vi "En Face Functional Global.vi"(8 "Error In":errorcluster, 10 "BScan Index":dbl, 11 "Input":sgl[][](graph)) -> (0 "Error Out":errorcluster)   [LabVIEW 2015]
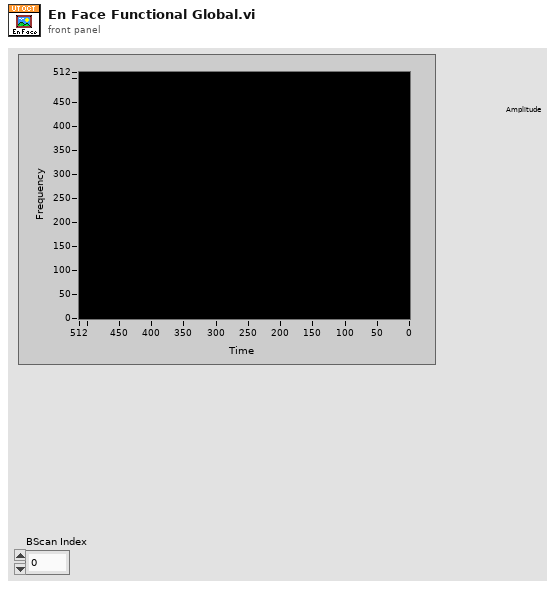
[diagram p1: front panel]
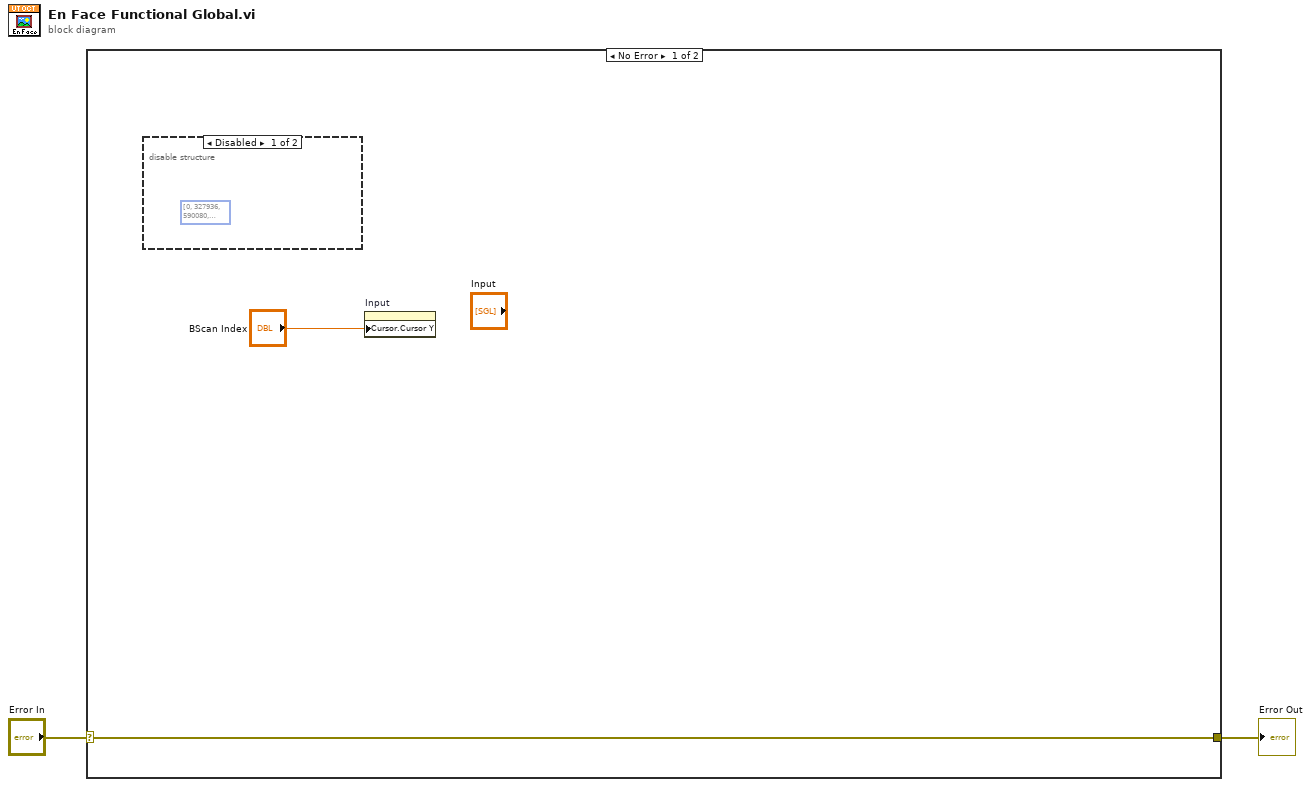
[diagram p0: block diagram]
diagram:
  n1 = case shown="No Error" "Error In" {
    selector: "Error In" -> [w4 w5]
    tunnel: [w4 w5] -> w1
    frame No Error {
      n2 = disable-structure shown="Disabled" {
        frame Disabled {
          (unwired) u32[] [0, 327936, 590080, 852224, 983296, 1114624, 1180160, 1311232, 1442304, 1573632, 1704704, 1770240, 1901312, 1966848, 2098176, 2163712, 2294784, 2491392, 2557184, 2688256, 2753792, 2884864, 2950656, 3081728, 3147264, 3344129, 3475457, 3540993, 3672321, 3738113, 3869185, 3934977, 4066305, 4197633, 4328961, 4394497, 4460289, 4591617, 4657409, 4788481, 4854273, 4985601, 5116929, 5248257, 5314049, 5379841, 5511169, 5576961, 5708033, 5773825, 5905153, 6036482, 6167810, 6233346, 6299138, 6430466, 6496258, 6562050, 6693634, 6759426, 6890754, 7022082, 7087874, 7153666, 7284994, 7350786, 7482114, 7547906, 7613698, 7745026, 7876354, 8007682, 8073474, 8139522, 8205314, 8336642, 8467970, 8533763, 8599555, 8665347, 8731139, 8862467, 8993795, 9059587, 9125380, 9191428, 9257220, 9388548, 9454340, 9520132, 9585924, 9717253, 9848837, 9914629, 9980165, 10045957, 10177541, 10243334, 10309126, 10375174, 10440966, 10572294, 10703623, 10769416, 10835208, 10901256, 10967049, 11033097, 11033609, 11099401, 11165450, 11231242, 11231754, 11297547, 11363339, 11429131, 11495180, 11495692, 11561740, 11693069, 11758861, 11759373, 11825165, 11891214, 11957006, 12022799, 12023311, 12089103, 12220944, 12286736, 12286736, 12352529, 12418577, 12484370, 12550162, 12615954, 12681747, 12747796, 12813588, 12813845, 12879894, 12945686, 13077015, 13142808, 13143064, 13208856, 13274905, 13340697, 13340953, 13472282, 13538075, 13604379, 13670172, 13735964, 13801757, 13867550, 13933343, 13999392, 13999648, 14065441, 14131234, 14197027, 14197541, 14263334, 14329383, 14395176, 14460969, 14592553, 14658346, 14724139, 14789932, 14790189, 14856238, 14922287, 14988080, 15053873, 15054130, 15119923, 15185972, 15251765, 15317559, 15383353, 15449146, 15449660, 15515454, 15515968, 15516226, 15582021, 15582278, 15582536, 15648587, 15648844, 15714639, 15714897, 15715155, 15780949, 15781463, 15847256, 15847770, 15848028, 15913823, 15914081, 15979875, 15980133, 15980391, 16046441, 16046444, 16046703, 16046705, 16112500, 16113015, 16113274, 16113277, 16179072, 16179330, 16179588, 16245384, 16245387, 16245389, 16245648, 16311443, 16376982, 16377241, 16377499, 16443294, 16443553, 16443555, 16443815, 16509866, 16510124, 16510127, 16575923, 16575924, 16576182, 16576441, 16576443, 16576702, 16576705, 16576963, 16577222, 16577224, 16577482, 16577485, 16577743, 16577745, 16578004, 16578262, 16578264, 16578523, 16578782, 16579040, 16579299, 16579301, 16579303, 16579562, 16579821] ("Color Table")
        }
        frame Enabled {
        }
      }
      n3 = property on="Input" class="IntGraph (strict)"("Cursor.Cursor Y"="BScan Index") -> ()  [unwired: 2 in, 2 out]
    }
    frame Error {
    }
  }
  "Error Out" <- w1
